vi "Bertta_v07.vi"() -> ()   [LabVIEW 2015]
uses:
  x64/Debug/BERTTA.dll
panel:
  in  "OK Button":bool
  in  "Tab Control":T1(tab)
  in  "Description":string
  in  "Project name":string
  in  "User (initials)":string
  out "PUMP 1":bool
  out "Target amount":dbl
  out "Scale weight":dbl
  out "Amount now":dbl
  out "Flow rate":dbl
  out "Time to target":dbl format="%<%H:%M:%S>t"
  out "Current step":dbl
  out "Target amount":dbl
  out "Amount now":dbl
  out "Tr":dbl
  out "Tj in":dbl
  out "Tj out":dbl
  out "T init":dbl
  out "T set":dbl
  out "Current step":i32
  out "RPM":dbl
  out "Torque 2":dbl
  out "Waveform Chart 5":dynamicdata(graph)
  out "Waveform Chart 6":dynamicdata(graph)
  out "Waveform Chart 7":dynamicdata(graph)
  in  "Signals":bool[](array[boolean])
  out "Waveform Chart 3":dynamicdata(graph)
  out "Table":string[][](table)
  in  "Headers":string[](array[string])
  out "Boolean 12":bool
  out "Boolean 7":bool
  out "Boolean 6":bool
  out "Boolean 5":bool
  out "Boolean 4":bool
  in  "?":bool
  in  "Seq":dbl[][](array[numeric])=[[20.0, 45.0, 50.0], [46.0, 50.0, 20.0], [3.0, 3.0, 3.0]]
  out "T control":dbl
  out "Tr":dbl
  out "Tj in":dbl
  out "Tj out":dbl
  out "DT":dbl
  out "Current step":i32
  out "Elapsed":i32
  in  "Tbypass":dbl=20.0
  in  "Tfail":dbl=22.0
  in  "err":i32
  in  "PAUSE":bool
  out "Tinit":dbl
  out "Tset":dbl
  out "Time limit":dbl
  out "Waveform Chart":dynamicdata(graph)
  in  "Lauda port":dbl=9.0
  out "Data out":dbl
  out "Data out":dbl
  in  "Port":i32=10
  in  "Radio Buttons":enum32{"Reglo Digital", "Reglo Analog", "PAM"}(radio)
  out "Speed":dbl
  out "mA":dbl format="%#_2g"
  in  "Port":i32=15
  out "RPM":dbl format="%#_2g"
  out "Boolean 18":bool
  out "Boolean 17":bool
  out "Boolean 16":bool
  out "Boolean 15":bool
  out "Boolean 14":bool
  out "Boolean 13":bool
  out "Boolean 11":bool
  out "Boolean 10":bool
  out "Boolean 9":bool
  out "Boolean 8":bool
  in  "Seq 2":dbl[][](array[numeric])=[[3.0, 3.0, 7.0], [2.0, 2.0, 2.0], [4.0, 2.0, 100.0]]
  in  "?":bool
  out "Flow rate (g/min)":dbl
  out "Time (min)":dbl
  out "Target (g)":dbl
  out "Scale reading":dbl
  out "Step amount now":dbl
  out "Time to target":dbl format="%<%H:%M:%S>t"
  in  "Bypass (g/min)":dbl
  out "Waveform Chart 2":dynamicdata(graph)
  in  "?":bool
  out "Total amount now":dbl
  out "Total time":dbl
  out "Total amount target":dbl
  out "RPM":dbl
  out "Torque":dbl
  in  "Set RPM":dbl(slide) scale=0.0..500.0
  out "Waveform Chart 4":dynamicdata(graph)
  in  "?":T2(tab)
  in  "Device port":dbl=13.0
  # "PUMP & SCALE 1"
  # "STEP"
  # "TOTAL"
  # "Flow rate (P1)"
  # "Scale 1 weight"
  # "Amount / step (P1)"
  # "Step (P1)"
  # "T control"
  # "Tj in"
  # "Tj out"
  # "Tr"
  # "RPM"
  # "Torque"
  # "Tinit     >    Tset       min. time"
  # "Grams    /   min"
  # "Pump configuration"
  # "Scale configuration"
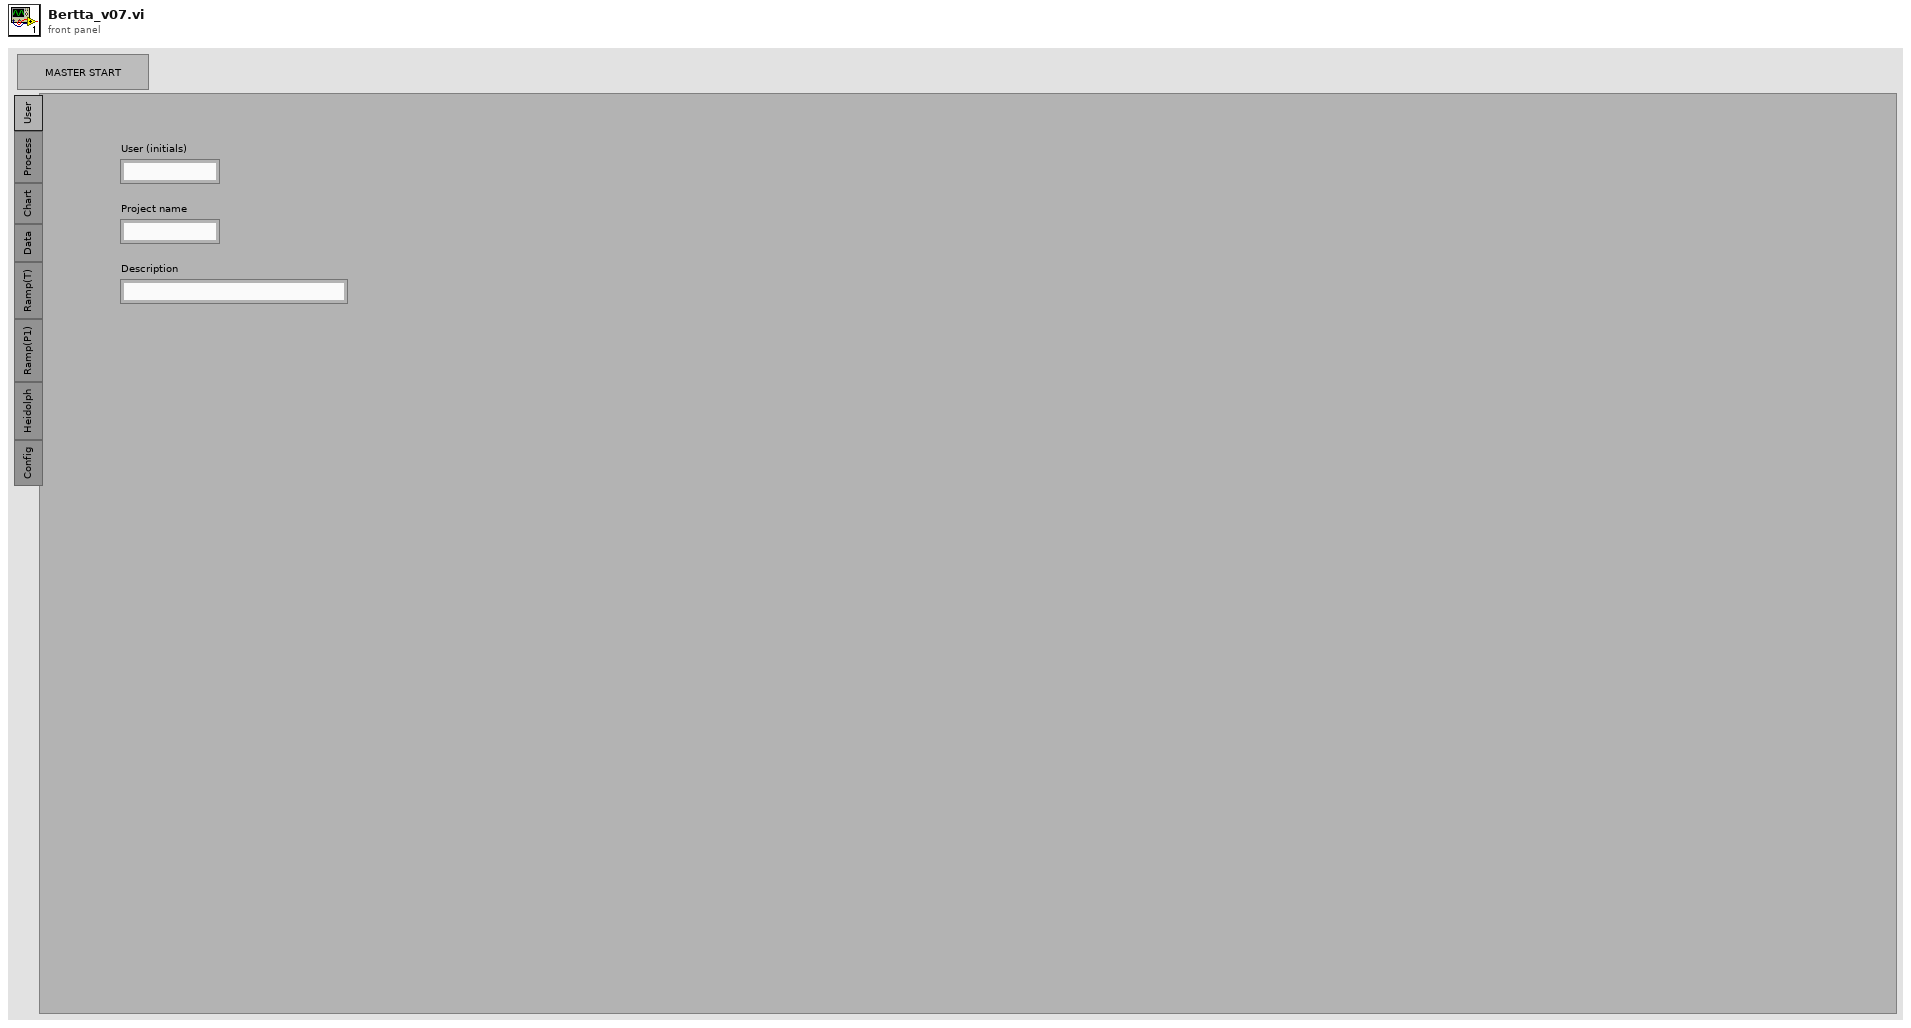
[diagram p1: front panel]
types:
  T1 = enum32{"User", "Process", "Chart", "Data", "Ramp(T)", "Ramp(P1)", "Heidolph", "Config"}
  T2 = enum32{"DB / File", "Lauda", "Heidolph", "Mettler 1", "Mettler 2", "Mettler 3", "Ismatec 1"}
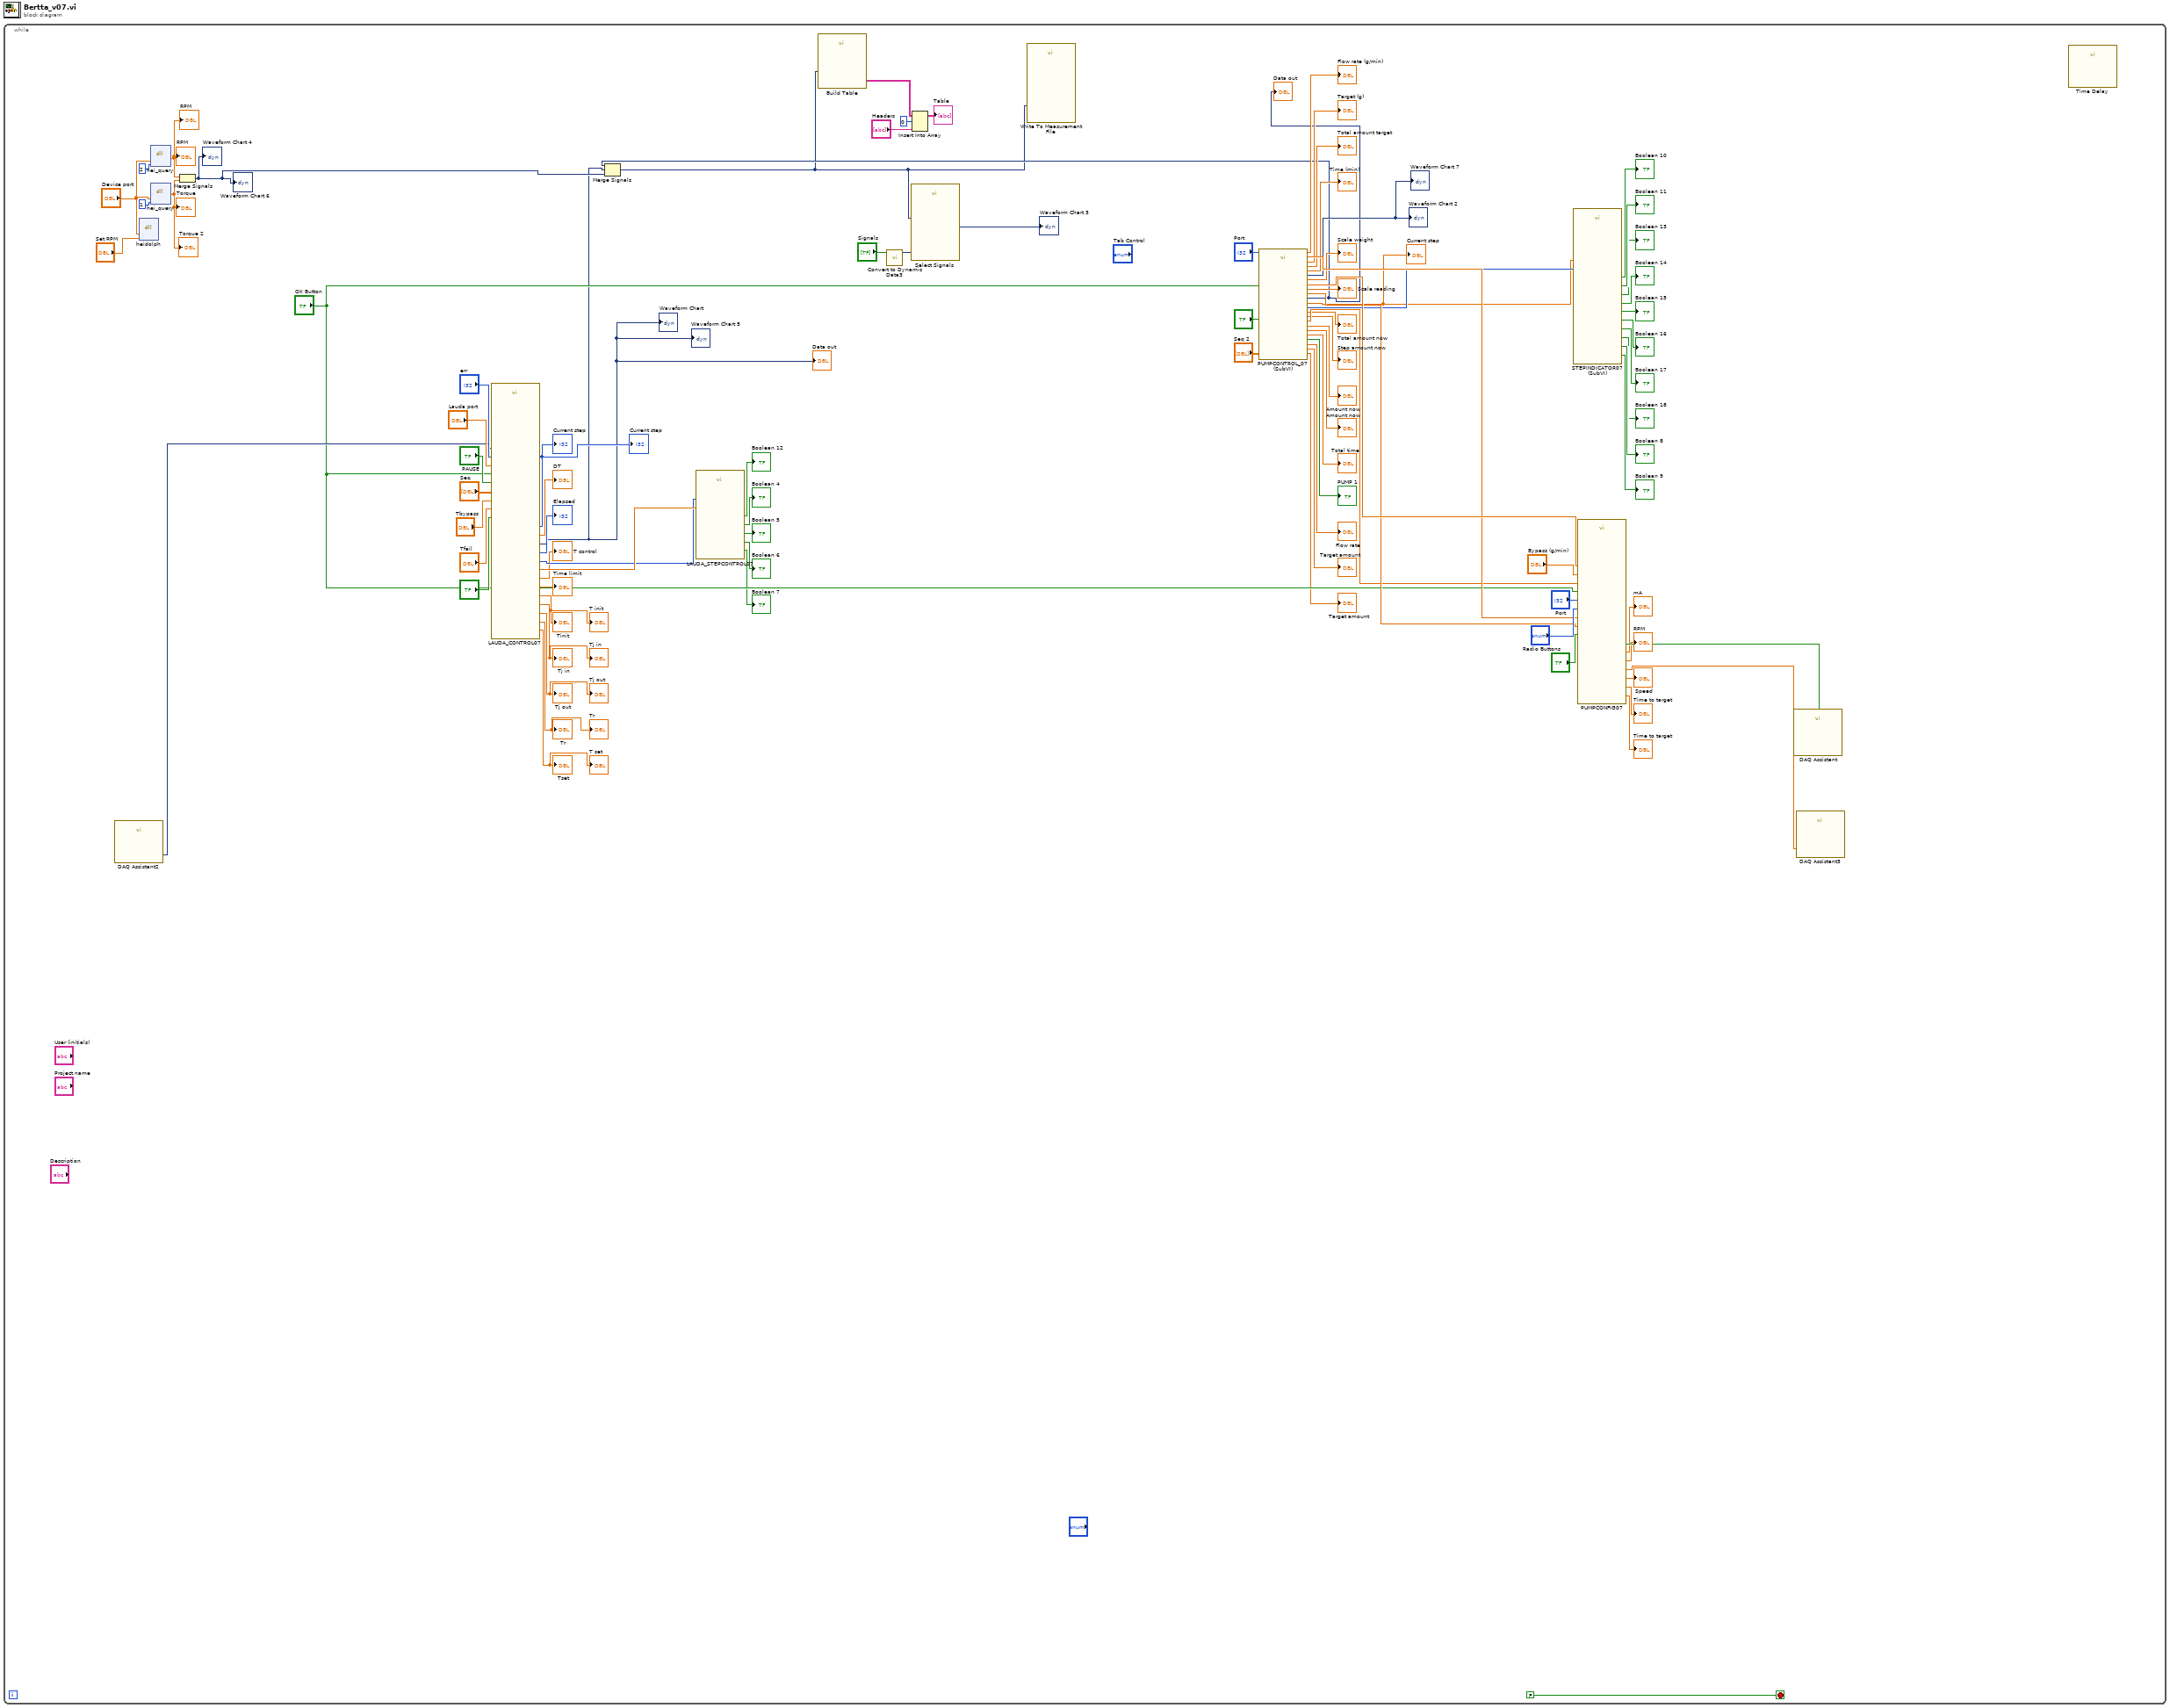
[diagram p0: block diagram]
diagram:
  n1 = while {
    stop <- FALSE stop-if-true
    n2 = call "DAQ Assistant2"() -> ("data"=w65:dynamicdata)  [unwired: 17 in, 2 out]
    n3 = dll-call lib="C:/Users/shresplab/OneDrive - Kemira Oyj/Documents/Visual Studio 2017/Projects/Bertta/BERTTA/x64/Debug/BERTTA.dll" fn="heidolph"("port"="Device port", "speed"="Set RPM") -> ()  [unwired: 6 in, 2 out]
    n4 = dll-call lib="C:/Users/shresplab/OneDrive - Kemira Oyj/Documents/Visual Studio 2017/Projects/Bertta/BERTTA/x64/Debug/BERTTA.dll" fn="hei_query"("port"="Device port", "q"=2) -> ("return type"=w7:dbl)  [unwired: 5 in, 2 out]
    "RPM" <- w7
    "RPM" <- w7
    n5 = dll-call lib="C:/Users/shresplab/OneDrive - Kemira Oyj/Documents/Visual Studio 2017/Projects/Bertta/BERTTA/x64/Debug/BERTTA.dll" fn="hei_query"("port"="Device port", "q"=1) -> ("return type"=w6:dbl)  [unwired: 5 in, 2 out]
    "Torque" <- w6
    "Torque 2" <- w6
    n6 = Merge Signals(w7, w6) -> (w5:dynamicdata)
    "Waveform Chart 4" <- w5
    "Waveform Chart 6" <- w5
    n7 = call "LAUDA_CONTROL07.vi"(0:"?", "PAUSE"="PAUSE", "data"=w65, "Seq"="Seq", "Lauda port"="Lauda port", "Tbypass"="Tbypass", "Tfail"="Tfail", "err"="err", "OK Button"="OK Button") -> (12:"Tj out"=→"Tj in" →"Tj in":dbl, "DT"=→"DT":dbl, 16:"Tj out"=→"Tj out" →"Tj out":dbl, "Tset"=→"Tset" →"T set":dbl, "Dynamic Data"=w3:dynamicdata, "Time limit"=→"Time limit":dbl, "Numeric"=w72:i16, "Numeric 2"=w73:dbl, "T control"=→"T control":dbl, "Current step"=→"Current step" →"Current step":i32, "Elapsed"=→"Elapsed":i32, "Tr"=→"Tr" →"Tr":dbl, "Tinit"=→"Tinit" →"T init":dbl)  [unwired: 6 in]
    "Waveform Chart" <- w3
    "Data out" <- w3
    "Waveform Chart 5" <- w3
    n8 = call "LAUDA_STEPCONTROL07.vi"("Numeric 2"=w73, "Numeric"=w72) -> ("Boolean 6"=→"Boolean 6":bool, "Boolean 5"=→"Boolean 5":bool, "Boolean 4"=→"Boolean 4":bool, "Boolean 7"=→"Boolean 7":bool, "Boolean 12"=→"Boolean 12":bool)  [unwired: 5 in]
    n9 = call "Convert to Dynamic Data3"("Array"="Signals") -> ("Dynamic Data Type"=w84:dynamicdata)  [unwired: 3 in]
    n10 = call "PUMPCONTROL_07 (SubVI).vi"("Port"="Port", "OK Button"="OK Button", 2:"?", "Seq in"="Seq 2") -> ("Amount now"=→"Amount now":dbl, "Amount now 2"=→"Amount now":dbl, "Flow rate out"=w55:dbl, "Step amount now"=→"Step amount now":dbl, "Total amount now"=→"Total amount now":dbl, "Total time"=→"Total time":dbl, "Numeric 2"=w61:i16, "PUMP 1"=→"PUMP 1":bool, "Numeric"=w54:dbl, "Flow rate"=→"Flow rate":dbl, "Dynamic Data"=w4:dynamicdata, "Target amount"=→"Target amount":dbl, "Time (min) 2"=w62:dbl, "Target amount 2"=→"Target amount":dbl, "Scale reading"=→"Scale reading":dbl, "Flow rate (g/min)"=→"Flow rate (g/min)":dbl, "Target (g) 2"=w63:dbl, "Target (g)"=→"Target (g)":dbl, "Total amount target"=→"Total amount target":dbl, "Time (min)"=→"Time (min)":dbl, "Waveform Chart 2"=→"Waveform Chart 2" →"Waveform Chart 7":dynamicdata, "Scale weight"=→"Scale weight":dbl, "Amount (g)"=w64:dbl)  [unwired: 1 in]
    "Current step" <- w54
    "Data out" <- w4
    n11 = Merge Signals(w4, w3, w5) -> (w1:dynamicdata)
    n12 = call "Build Table"("Signals"=w1) -> ("Table"=w86:string[][])  [unwired: 4 in, 6 out]
    n13 = call "Select Signals"("Selector Input"=w84, "Signals"=w1) -> ("Signal Out"=→"Waveform Chart 3":dynamicdata)  [unwired: 8 in, 1 out]
    n14 = Insert Into Array(array=w86, index (row)=0, new element="Headers") -> (→"Table":string[][])  [unwired: 1 in]
    n15 = call "Write To Measurement File"("Signals"=w1) -> ()  [unwired: 16 in, 3 out]
    n16 = call "STEPINDICATOR07 (SubVI).vi"("Numeric"=w54, "Numeric 2"=w61) -> ("Boolean 18"=→"Boolean 18":bool, "Boolean 8"=→"Boolean 8":bool, "Boolean 9"=→"Boolean 9":bool, "Boolean 17"=→"Boolean 17":bool, "Boolean 10"=→"Boolean 10":bool, "Boolean 16"=→"Boolean 16":bool, "Boolean 11"=→"Boolean 11":bool, "Boolean 15"=→"Boolean 15":bool, "Boolean 14"=→"Boolean 14":bool, "Boolean 13"=→"Boolean 13":bool)  [unwired: 4 in]
    n17 = call "PUMPCONFIG07.vi"(0:"?", "Radio Buttons"="Radio Buttons", "Bypass (g/min)"="Bypass (g/min)", "Target (g) in"=w63, "Amount (g)"=w64, "Time (min) in"=w62, "Flow rate in"=w55, "OK Button"="OK Button", "Port"="Port") -> ("Time to target 2"=→"Time to target":dbl, "Time to target"=→"Time to target":dbl, "mA"=→"mA":dbl, "signal"=w70:dbl, "Speed"=→"Speed":dbl, "RPM"=→"RPM":dbl, "Array"=w71:bool[])
    n18 = call "DAQ Assistant"("data"=w71) -> ()  [unwired: 17 in, 2 out]
    n19 = call "DAQ Assistant3"("data"=w70) -> ()  [unwired: 17 in, 2 out]
    n20 = call "Time Delay"() -> ()  [unwired: 11 in, 1 out]
  }
